vi "Check Not Stopped Streaming.vi"(8 "error in (no error)":errorcluster, 11 "Camera in":refnum<class "Camera.lvclass">) -> (0 "error out":errorcluster)   [LabVIEW 2020, in "Camera.lvclass"]
uses:
  Camera.lvclass
  Camera.lvclass/Camera.ctl
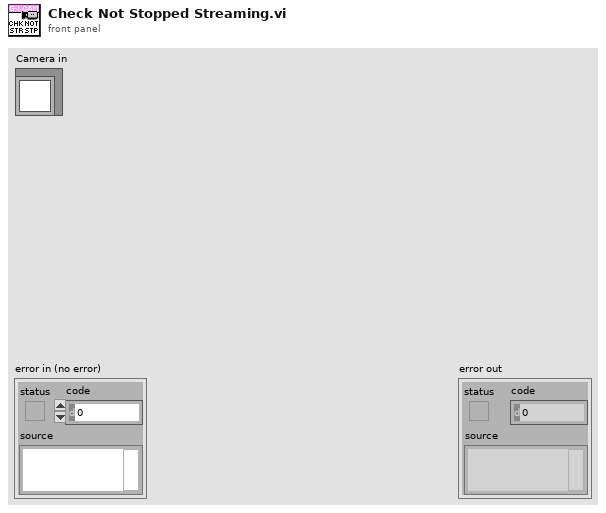
[diagram p1: front panel]
types:
  T1 = typedef "Camera.lvclass/Streaming Registation.ctl" = cluster{"Streaming Stopped":refnum<event-registration>, "User Event":refnum<user-event>}
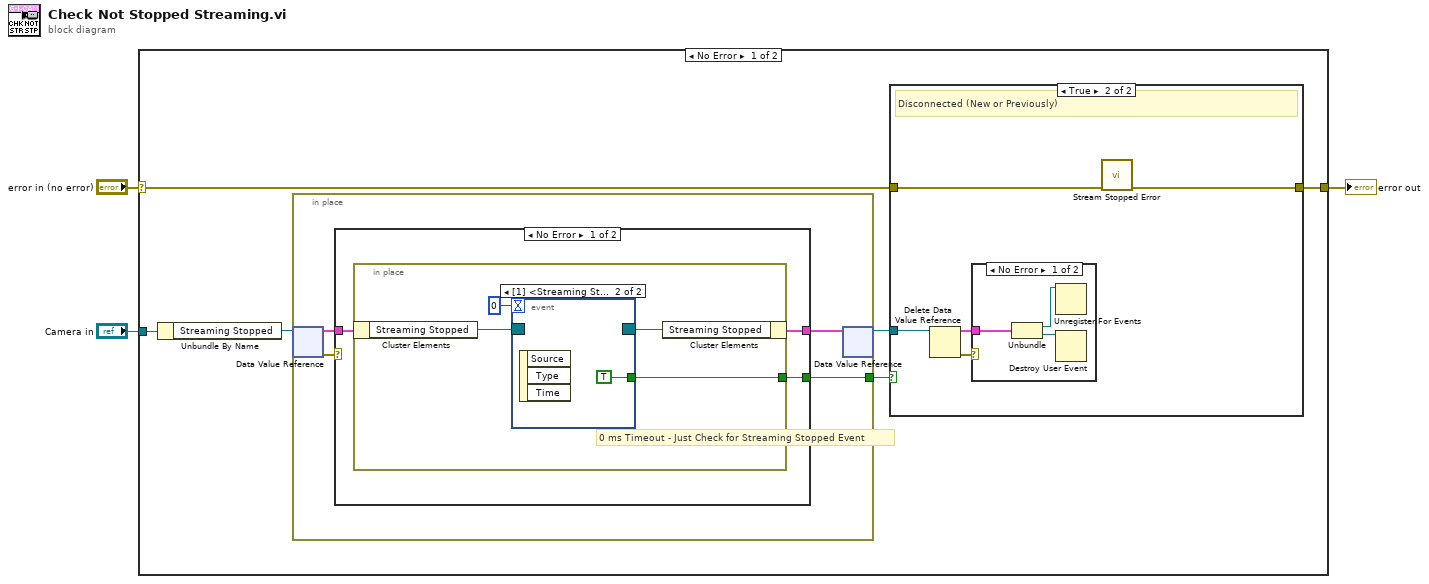
[diagram p0: block diagram]
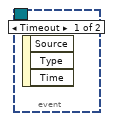
[diagram p4: hidden frame]
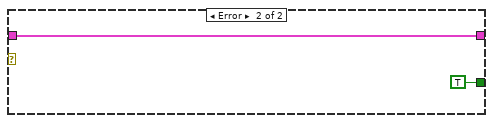
[diagram p5: hidden frame]
diagram:
  n1 = case shown="No Error" "error in (no error)" {
    selector: "error in (no error)" -> [w6 w33]
    tunnel: [w5 w33] -> w2
    tunnel: "Camera in" -> [w9 _]
    frame No Error {
      n2 = Unbundle By Name(w9) -> ("Streaming Stopped"=w8:refnum<data-value>)
      n3 = in-place {
        in-place-border: [w19] -> w7
        n4 = in-place-dvr #1(w8) -> (w21:T1, w22:errorcluster)
        n5 = case shown="No Error" w22 {
          tunnel: w21 -> [w24 w31]
          tunnel: [w23 w31] -> w20
          tunnel: [w25 TRUE] -> w19
          frame No Error {
            n6 = in-place {
              in-place-border: [w28] -> w25
              # "0 ms Timeout - Just Check for Streaming Stopped Event"
              n7 = in-place-cluster #2(w24) -> ("Streaming Stopped"=w27:refnum<event-registration>)
              n8 = event shown="[1] <Streaming Stopped>: User Event" {
                selector: w27 -> [_ _]
                dyn-events: [_ _] -> w26
                timeout: 0 -> [_ _]
                tunnel: [_ TRUE] -> w28
                event Timeout {
                  n9 = event-data() -> ()  [unwired: 1 in, 3 out]
                }
                event User Event {
                  n10 = event-data() -> ()  [unwired: 1 in, 3 out]
                }
              }
              n11 = in-place-cluster #2("Streaming Stopped"=w26) -> (w23:T1)
            }
          }
          frame Error {
          }
        }
        n12 = in-place-dvr #1(w20) -> (w4:refnum<data-value>)  [unwired: 1 out]
      }
      n13 = case shown="True" w7 {
        tunnel: w6 -> [w10 w15]
        tunnel: [w10 w14] -> w5
        tunnel: w4 -> [_ w13]
        frame False {
          # "Still Connected"
        }
        frame True {
          # "Disconnected (New or Previously)"
          n14 = Delete Data Value Reference(data value reference=w13) -> (data value=w12:T1, error out=w11:errorcluster)  [unwired: 1 in]
          n15 = case shown="No Error" w11 {
            tunnel: w12 -> [w18 _]
            frame No Error {
              n16 = Unbundle(w18) -> ("Streaming Stopped"=w17:refnum<event-registration>, "User Event"=w16:refnum<user-event>)
              n17 = Unregister For Events(event registration refnum=w17) -> ()  [unwired: 1 in, 1 out]
              n18 = Destroy User Event(user event=w16) -> ()  [unwired: 1 in, 1 out]
            }
            frame Error {
            }
          }
          n19 = call "Stream Stopped Error.vi"("error in (no error)"=w15) -> ("error out"=w14:errorcluster)  [unwired: 10 in]
        }
      }
    }
    frame Error {
    }
  }
  "error out" <- w2
